vi "odd_even_setup.vi"(9 "Num. of Drops in":dbl, 10 "Pitch in":dbl[](array[numeric]), 11 "Distance b/w cells in":dbl[](array[numeric])) -> ()   [LabVIEW 2021]
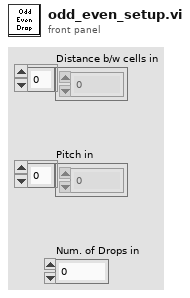
[diagram p1: front panel]
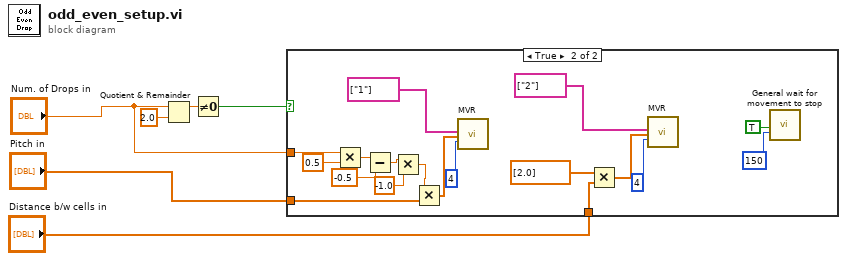
[diagram p0: block diagram]
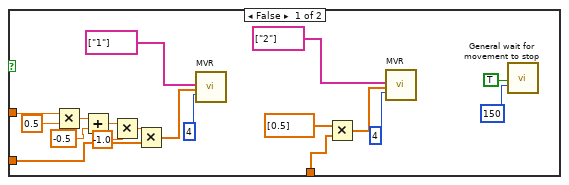
[diagram p2: hidden frame]
diagram:
  n1 = Quotient & Remainder(x="Num. of Drops in", y=2.0) -> (x-y*floor(x/y)=w3:dbl)  [unwired: 1 out]
  n2 = Not Equal To 0?(x=w3) -> (x != 0?=w4:bool)
  n3 = case shown="True" w4 {
    tunnel: "Pitch in" -> [w15 w40]
    tunnel: "Distance b/w cells in" -> [w14 w37]
    tunnel: "Num. of Drops in" -> [w12 w31]
    frame False {
      n4 = Multiply(x=w12, y=0.5) -> (x*y=w11:dbl)
      n5 = Add(x=w11, y=-0.5) -> (x+y=w9:dbl)
      n6 = Multiply(x=w9, y=-1.0) -> (x*y=w7:dbl)
      n7 = Multiply(x=w7, y=w15) -> (x*y=w22:dbl[])
      n8 = call "MVR.vi"("Axes to move"=string[] ["1"], "Position values"=w22, "No.of digits"=i16 4) -> ()  [unwired: 2 in, 15 out]
      n9 = Multiply(x=dbl[] [0.5], y=w14) -> (x*y=w19:dbl[])
      n10 = call "MVR.vi"("Axes to move"=string[] ["2"], "Position values"=w19, "No.of digits"=i16 4) -> ()  [unwired: 2 in, 15 out]
      n11 = call "General wait for movement to stop.vi"("All axes?"=TRUE, "Additional wait time, ms"=u32 150) -> ()  [unwired: 6 in, 12 out]
    }
    frame True {
      n12 = Multiply(x=w31, y=0.5) -> (x*y=w29:dbl)
      n13 = Subtract(x=w29, y=-0.5) -> (x-y=w27:dbl)
      n14 = Multiply(x=w27, y=-1.0) -> (x*y=w25:dbl)
      n15 = Multiply(x=w25, y=w40) -> (x*y=w39:dbl[])
      n16 = call "MVR.vi"("Axes to move"=string[] ["1"], "Position values"=w39, "No.of digits"=i16 4) -> ()  [unwired: 2 in, 15 out]
      n17 = Multiply(x=dbl[] [2.0], y=w37) -> (x*y=w35:dbl[])
      n18 = call "MVR.vi"("Axes to move"=string[] ["2"], "Position values"=w35, "No.of digits"=i16 4) -> ()  [unwired: 2 in, 15 out]
      n19 = call "General wait for movement to stop.vi"("All axes?"=TRUE, "Additional wait time, ms"=u32 150) -> ()  [unwired: 6 in, 12 out]
    }
  }
